vi "TestCloneAPI.vi"() -> ()   [LabVIEW 2014, in "FgenModule.lvlib"]
uses:
  FgenModule.lvlib
  TestInfo.ctl
  <userlib>/NIST/ModuleAdminLib/ModuleAdmin/ModuleAdmin.lvclass
  PublicAPI/Arguments/Broadcasts/clDidInit.ctl
  <userlib>/NIST/ModuleAdminLib/ModuleAdmin/ModuleAdmin.lvclass/ModuleAdmin.ctl
  PublicAPI/Arguments/Requests/clStopArgument.ctl
  <userlib>/NIST/ModuleAdminLib/ModuleAdmin/Accessors/Read CloneRegRef.vi
  <userlib>/NIST/ModuleAdminLib/CloneRegistration/CloneRegistration.lvclass
  FgenPlugins/FgenPluginBaseClass/FgenPluginsBase.lvclass
panel:
  in  "Reset":bool
  in  "Query ID":bool
  in  "btnInitialize":bool
  in  "btnConfigTrigs":bool
  in  "btnGetWfrms":bool
  out "Waveform Chart":waveform(dbl)[](graph)=[{"t0"=timestamp(0 s since 1904-01-01), "dt"=0.00020833333333333335, "Y"=[0.0, 0.06540312923014306, 0.13052619222005157, 0.19509032201612825, 0.25881904510252074, 0.32143946530316153, 0.3826834323650897, 0.44228869021900125, 0.49999999999999994, 0.5555702330196022, 0.6087614290087205, 0.6593458151000688, 0.7071067811865475, 0.7518398074789774, 0.793353340291235, 0.8314696123025452, 0.8660254037844385, 0.8968727415326883, 0.9238795325112866, 0.9469301294951056, 0.9659258262890682, 0.9807852804032303, 0.9914448613738104, 0.9978589232386034, 1.0, 0.9978589232386034, 0.9914448613738104, 0.9807852804032303, 0.9659258262890683, 0.9469301294951056, 0.9238795325112868, 0.8968727415326883, 0.8660254037844388, 0.8314696123025452, 0.7933533402912354, 0.7518398074789774, 0.7071067811865478, 0.6593458151000688, 0.6087614290087209, 0.5555702330196023, 0.5000000000000002, 0.4422886902190014, 0.38268343236509, 0.32143946530316175, 0.258819045102521, 0.19509032201612847, 0.13052619222005185, 0.06540312923014331, 2.669170223387751e-16, -0.06540312923014278, -0.13052619222005132, -0.19509032201612794, -0.2588190451025205, -0.32143946530316125, -0.38268343236508956, -0.4422886902190009, -0.4999999999999998, -0.5555702330196018, -0.6087614290087204, -0.6593458151000685, -0.7071067811865474, -0.751839807478977, -0.793353340291235, -0.8314696123025449, -0.8660254037844386, -0.896872741532688, -0.9238795325112867, -0.9469301294951055, -0.9659258262890683, -0.9807852804032303, -0.9914448613738105, -0.9978589232386034, -1.0, -0.9978589232386034, -0.9914448613738105, -0.9807852804032303, -0.9659258262890684, -0.9469301294951056, -0.923879532511287, -0.8968727415326883, -0.8660254037844389, -0.8314696123025452, -0.7933533402912355, -0.7518398074789775, -0.7071067811865479, -0.6593458151000691, -0.6087614290087211, -0.5555702330196025, -0.5000000000000004, -0.44228869021900163, -0.3826834323650902, -0.321439465303162, -0.25881904510252124, -0.19509032201612872, -0.13052619222005207, -0.06540312923014356]}, {"t0"=timestamp(0 s since 1904-01-01), "dt"=0.00020833333333333335, "Y"=[-0.8660254037844387, -0.8968727415326884, -0.9238795325112867, -0.9469301294951057, -0.9659258262890682, -0.9807852804032304, -0.9914448613738103, -0.9978589232386035, -0.9999999999999999, -0.9978589232386035, -0.9914448613738103, -0.9807852804032304, -0.9659258262890681, -0.9469301294951056, -0.9238795325112865, -0.8968727415326883, -0.8660254037844384, -0.8314696123025451, -0.7933533402912349, -0.7518398074789773, -0.7071067811865474, -0.6593458151000687, -0.6087614290087205, -0.5555702330196021, -0.49999999999999994, -0.44228869021900113, -0.3826834323650897, -0.3214394653031614, -0.25881904510252074, -0.1950903220161281, -0.1305261922200516, -0.06540312923014292, -4.632253781944318e-17, 0.06540312923014319, 0.13052619222005152, 0.19509032201612836, 0.25881904510252063, 0.32143946530316164, 0.3826834323650896, 0.4422886902190013, 0.49999999999999983, 0.5555702330196022, 0.6087614290087204, 0.6593458151000688, 0.7071067811865474, 0.7518398074789774, 0.7933533402912349, 0.8314696123025452, 0.8660254037844384, 0.8968727415326883, 0.9238795325112865, 0.9469301294951056, 0.9659258262890681, 0.9807852804032303, 0.9914448613738103, 0.9978589232386034, 0.9999999999999999, 0.9978589232386034, 0.9914448613738103, 0.9807852804032303, 0.9659258262890682, 0.9469301294951056, 0.9238795325112867, 0.8968727415326883, 0.8660254037844387, 0.8314696123025452, 0.7933533402912353, 0.7518398074789774, 0.7071067811865477, 0.6593458151000688, 0.6087614290087209, 0.5555702330196022, 0.5000000000000002, 0.44228869021900125, 0.38268343236509, 0.3214394653031616, 0.258819045102521, 0.1950903220161283, 0.13052619222005188, 0.06540312923014313, 3.0540619946201053e-16, -0.06540312923014296, -0.13052619222005127, -0.19509032201612814, -0.2588190451025204, -0.3214394653031614, -0.3826834323650894, -0.4422886902190011, -0.4999999999999996, -0.555570233019602, -0.6087614290087202, -0.6593458151000686, -0.7071067811865471, -0.7518398074789772, -0.7933533402912348, -0.831469612302545]}, {"t0"=timestamp(0 s since 1904-01-01), "dt"=0.00020833333333333335, "Y"=[0.8660254037844387, 0.8314696123025455, 0.7933533402912353, 0.7518398074789776, 0.7071067811865477, 0.6593458151000691, 0.6087614290087209, 0.5555702330196024, 0.5000000000000002, 0.44228869021900147, 0.38268343236509, 0.3214394653031618, 0.258819045102521, 0.19509032201612853, 0.13052619222005188, 0.06540312923014334, 3.11409968992149e-16, -0.06540312923014278, -0.13052619222005127, -0.19509032201612797, -0.2588190451025204, -0.32143946530316125, -0.3826834323650894, -0.44228869021900097, -0.4999999999999996, -0.555570233019602, -0.6087614290087202, -0.6593458151000686, -0.7071067811865471, -0.7518398074789772, -0.7933533402912348, -0.831469612302545, -0.8660254037844384, -0.8968727415326881, -0.9238795325112865, -0.9469301294951056, -0.9659258262890681, -0.9807852804032304, -0.9914448613738103, -0.9978589232386035, -0.9999999999999999, -0.9978589232386035, -0.9914448613738104, -0.9807852804032304, -0.9659258262890683, -0.9469301294951057, -0.9238795325112868, -0.8968727415326884, -0.8660254037844388, -0.8314696123025453, -0.7933533402912354, -0.7518398074789776, -0.7071067811865478, -0.6593458151000692, -0.608761429008721, -0.5555702330196026, -0.5000000000000004, -0.44228869021900175, -0.3826834323650903, -0.3214394653031621, -0.2588190451025213, -0.1950903220161288, -0.13052619222005216, -0.06540312923014363, -5.937497672345304e-16, 0.06540312923014249, 0.130526192220051, 0.1950903220161277, 0.25881904510252013, 0.32143946530316103, 0.3826834323650891, 0.44228869021900075, 0.49999999999999933, 0.5555702330196017, 0.60876142900872, 0.6593458151000684, 0.7071067811865469, 0.7518398074789769, 0.7933533402912346, 0.8314696123025448, 0.8660254037844382, 0.8968727415326879, 0.9238795325112863, 0.9469301294951054, 0.9659258262890679, 0.9807852804032302, 0.99144486137381, 0.9978589232386034, 0.9999999999999998, 0.9978589232386035, 0.9914448613738103, 0.9807852804032305, 0.9659258262890683, 0.9469301294951058, 0.9238795325112868, 0.8968727415326886]}]
  in  "btnConfigFunc":bool
  in  "btnPref":bool
  in  "btnAbortGen":bool
  in  "btnInitiateGen":bool
  in  "Show Panel":bool=TRUE
  in  "Plugin Type":u16(ring) items=["DaqMx_Single", "Single_AM", "Base Plugin", "Agilent IVI FGen", "IVI Dual FGens", "IVI FGen", "Pxi6733_AM", "Pxi6733_Sine", "Pxi6733 Sine Standalone", "PMU Cal", "Test"]
  in  "btnLoadPlugin":bool
  out "Path":path
  in  "btnRequestINIPath":bool
  in  "btnRemove":bool
  out "Status Log":string
  out "Active Modules (Array)":string[](array[string])
  in  "btnAdd":bool
  in  "btnStop":bool
  in  "Select Module":i32(ring)=-1 caption="Select Module to send Request" items=["All"=-1, "4140002"=4140002]
  # "Hidden"
  # "Visible"
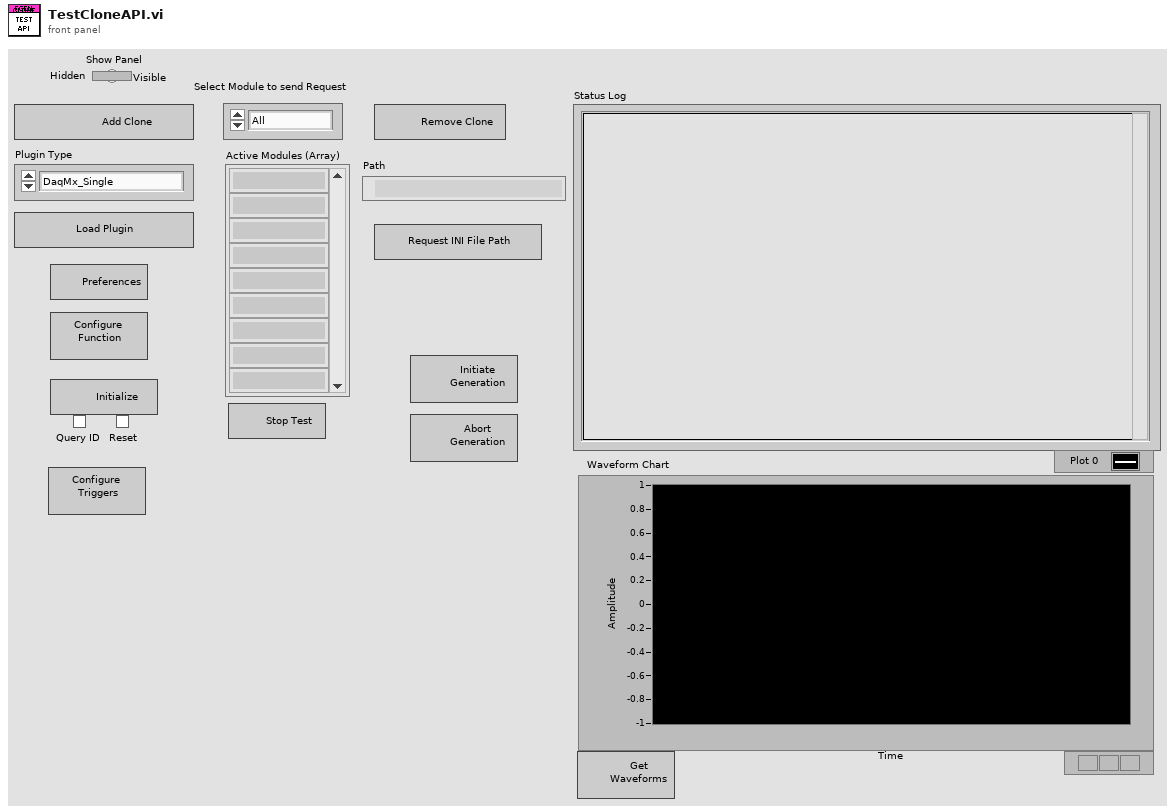
[diagram p1: front panel]
types:
  T1 = typedef "FgenModule.lvlib/TestInfo.ctl" = cluster{"PluginIniFilePaths":path[]}
  T2 = typedef "FgenModule.lvlib/clBroadcastEvents.ctl" = cluster{"DidInit":refnum<user-event>, "StatusUpdate":refnum<user-event>, "ErrorReport":refnum<user-event>, "DidStop":refnum<user-event>, "PathToINI":refnum<user-event>, "Channels":refnum<user-event>, "Function":refnum<user-event>, "Waveforms":refnum<user-event>, "Triggers":refnum<user-event>}
  T3 = typedef "FgenModule.lvlib/clDidInit.ctl" = cluster{"Init?":bool, "ModuleAdmin":refnum<class "ModuleAdmin.lvclass">}
  T4 = typedef "FgenModule.lvlib/clStopArgument.ctl" = cluster{"Exit via Stop Module Req?":bool, "Wait for Module to stop?":bool, "ModuleAdmin":refnum<class "ModuleAdmin.lvclass">}
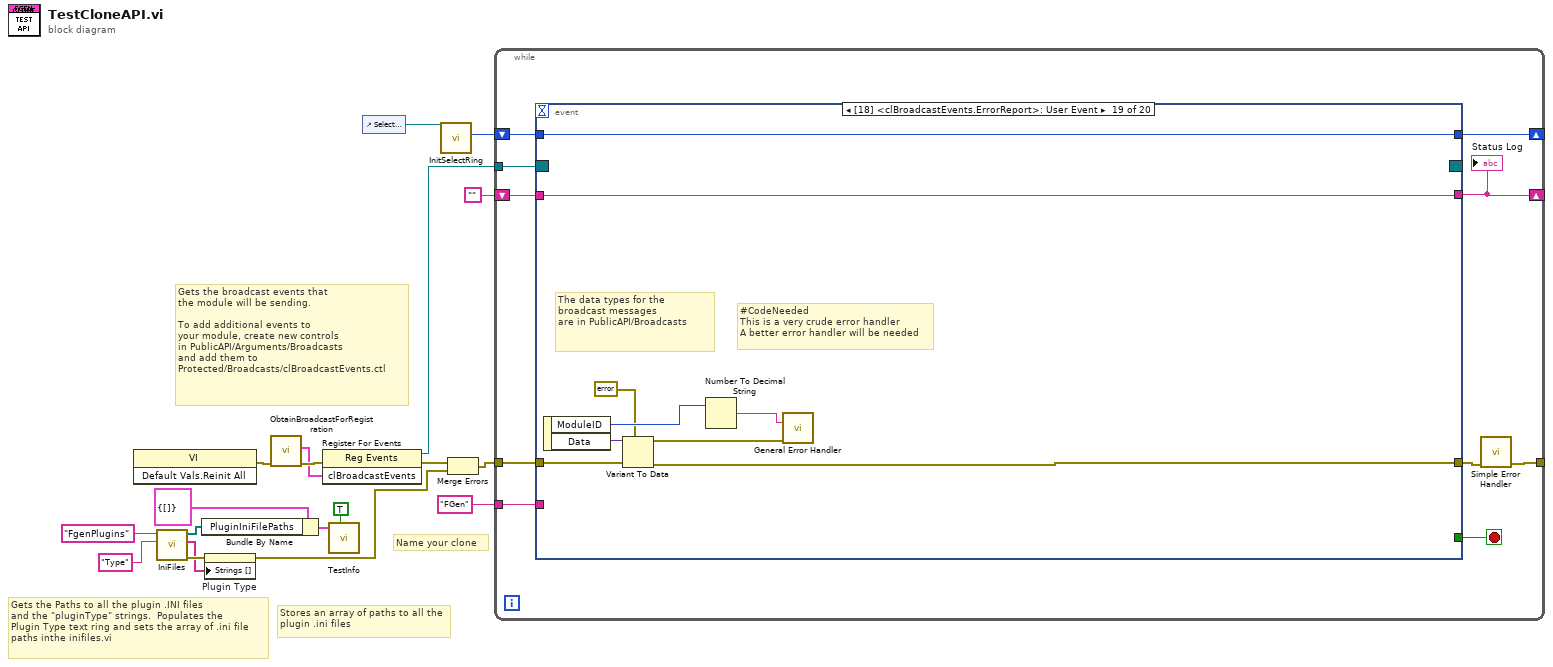
[diagram p0: block diagram]
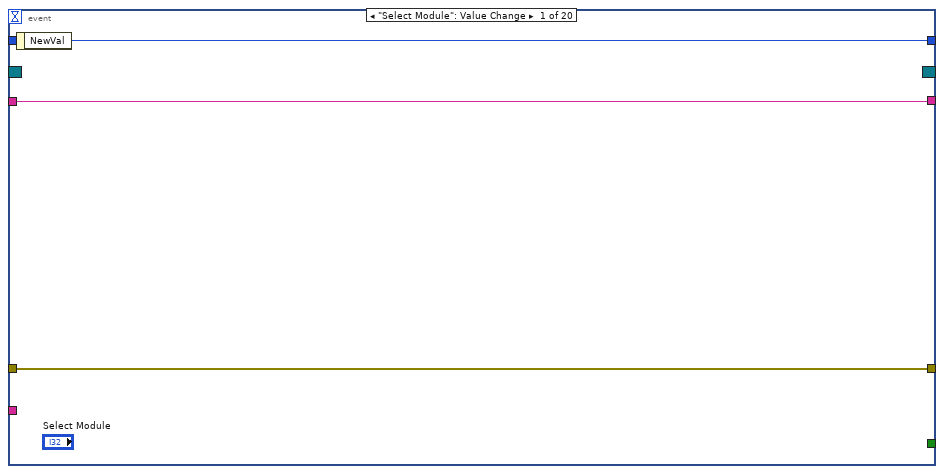
[diagram p2: hidden frame]
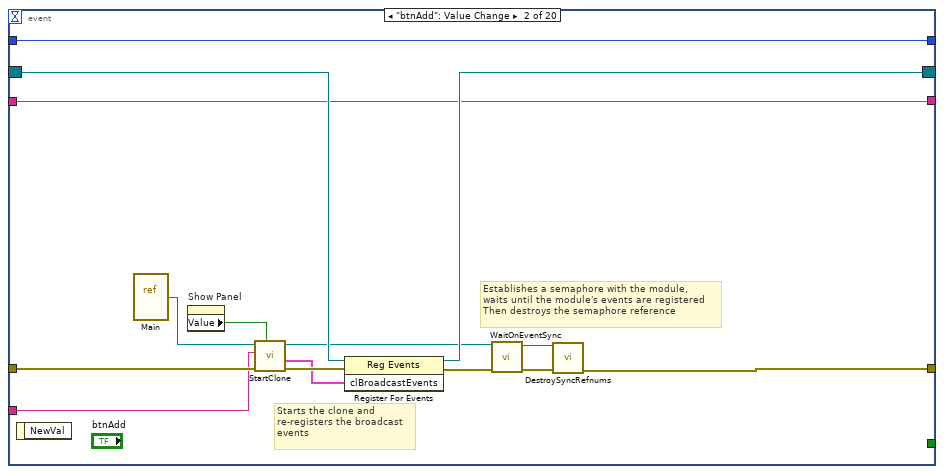
[diagram p3: hidden frame]
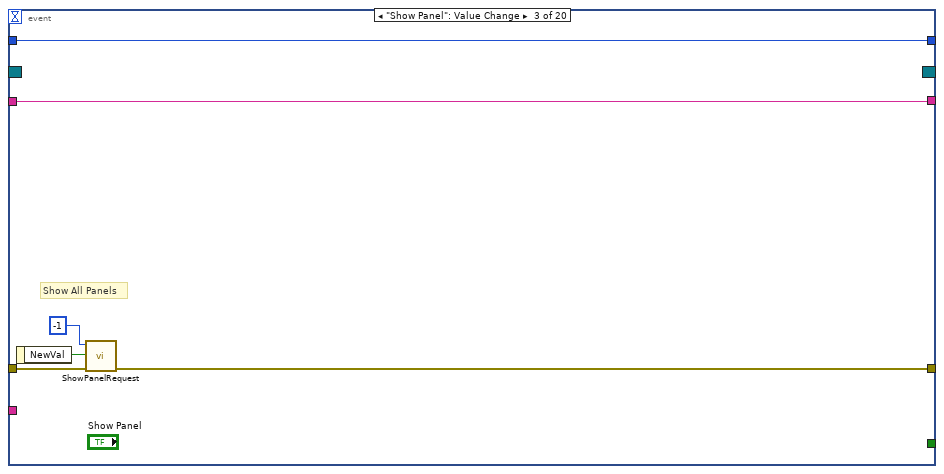
[diagram p4: hidden frame]
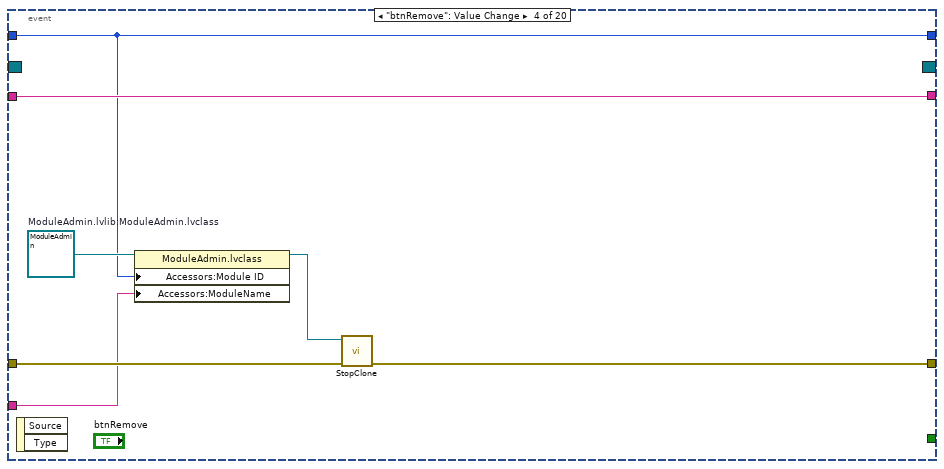
[diagram p5: hidden frame]
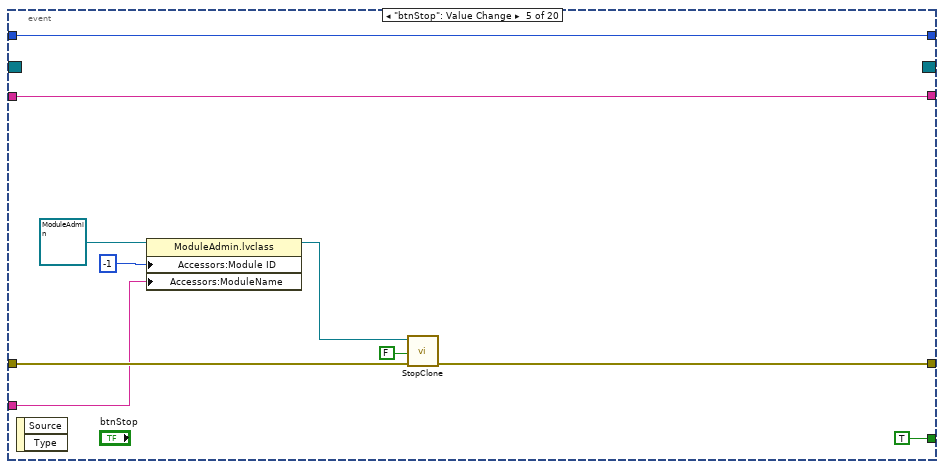
[diagram p6: hidden frame]
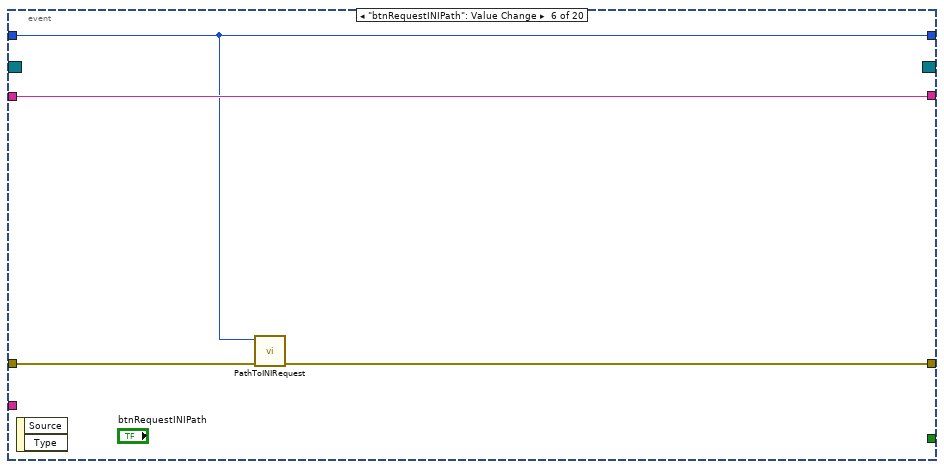
[diagram p7: hidden frame]
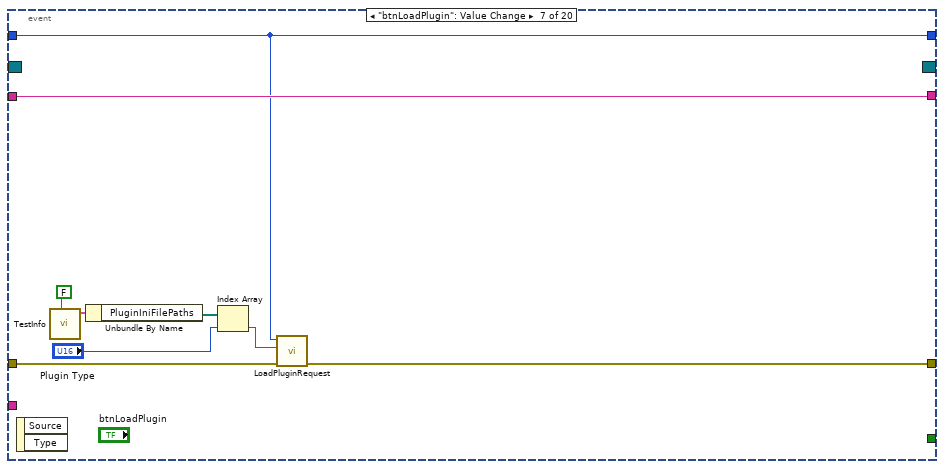
[diagram p8: hidden frame]
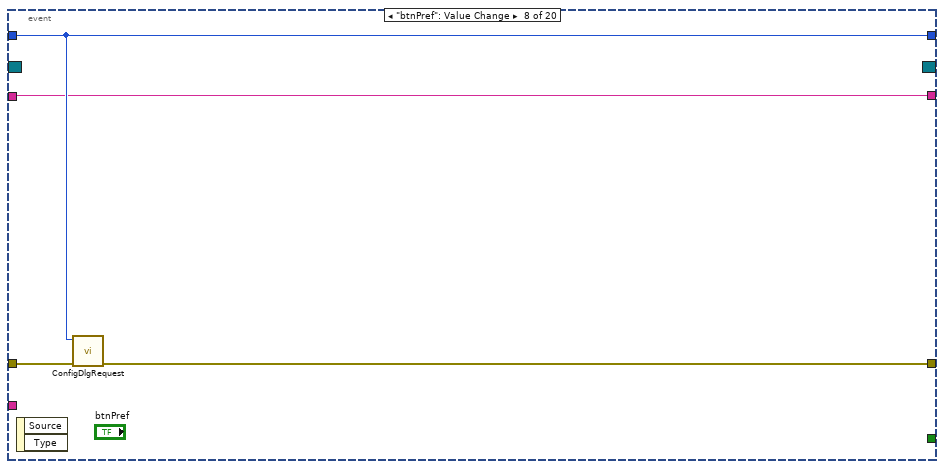
[diagram p9: hidden frame]
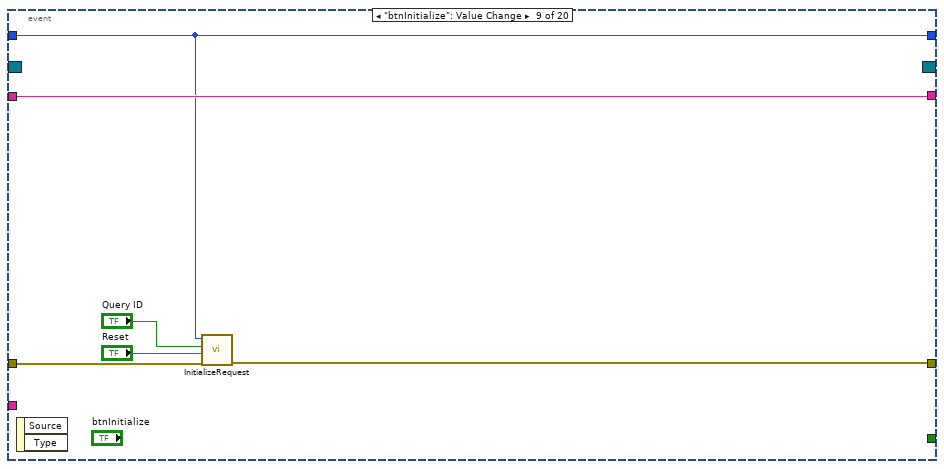
[diagram p10: hidden frame]
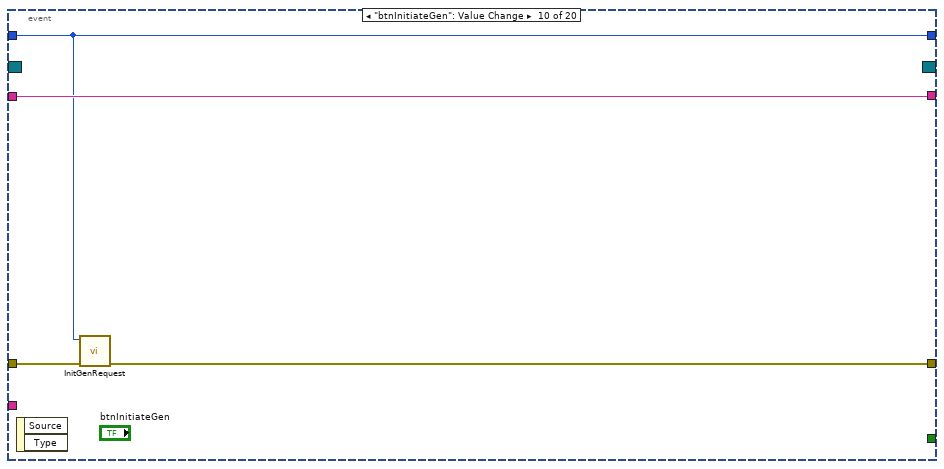
[diagram p11: hidden frame]
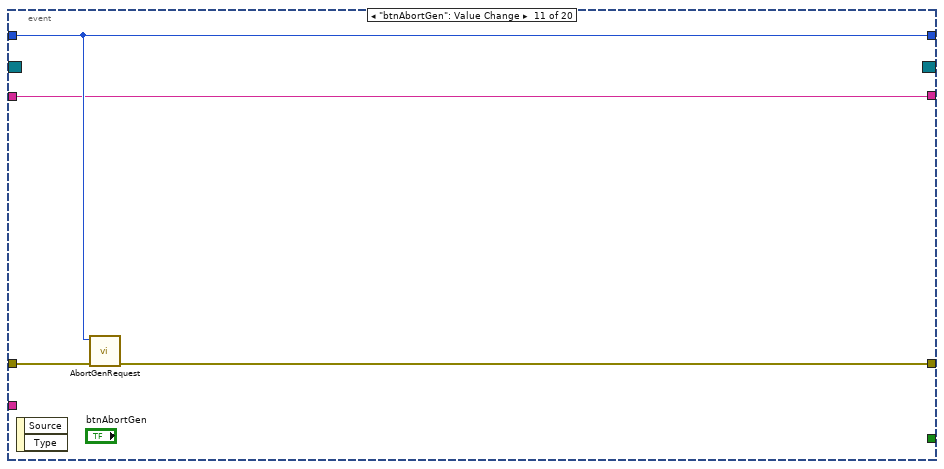
[diagram p12: hidden frame]
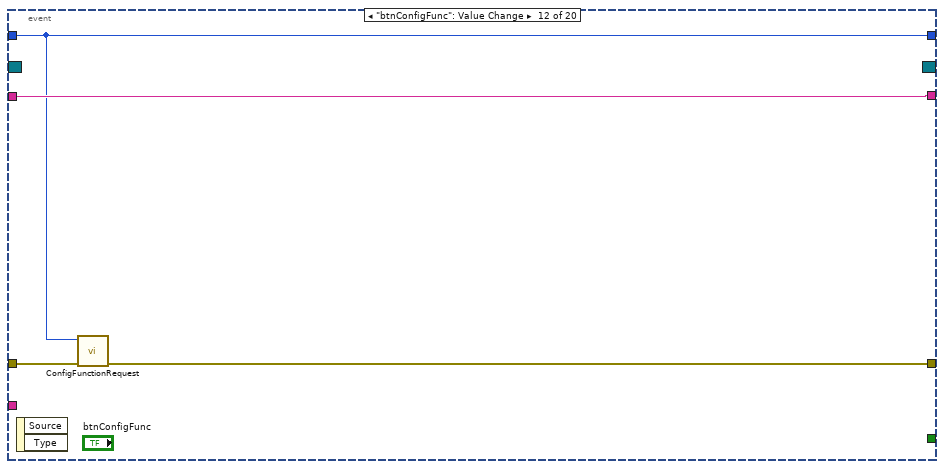
[diagram p13: hidden frame]
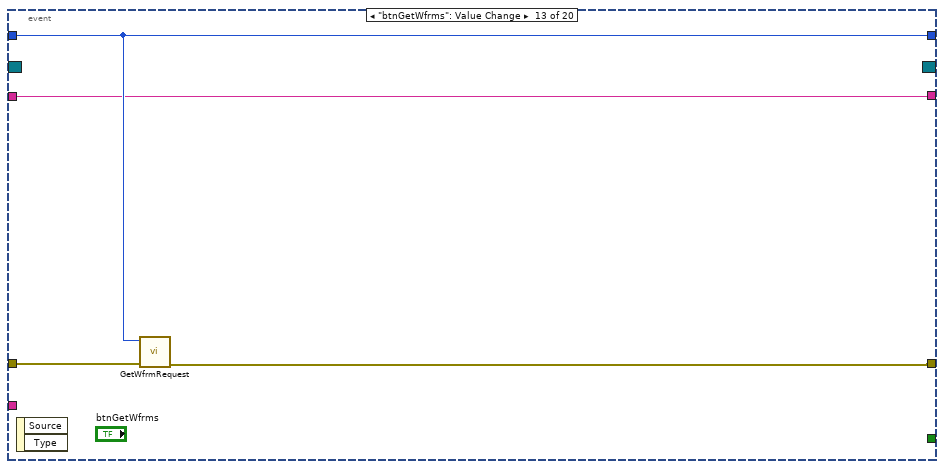
[diagram p14: hidden frame]
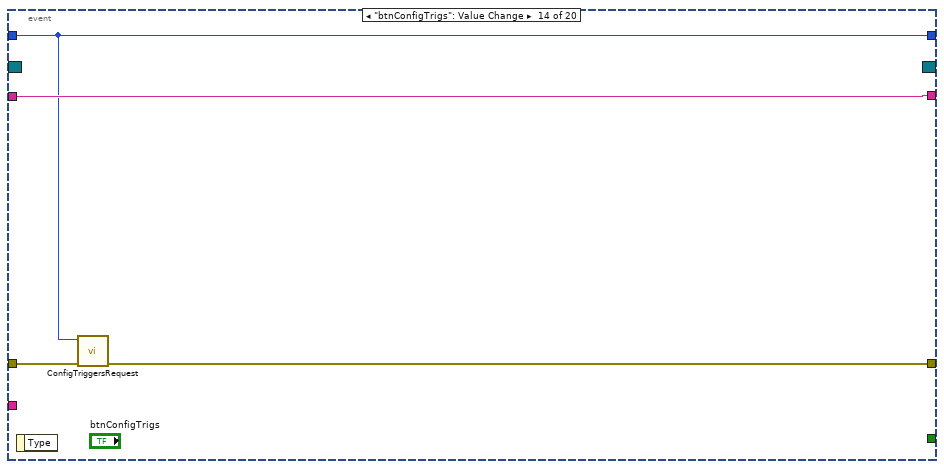
[diagram p15: hidden frame]
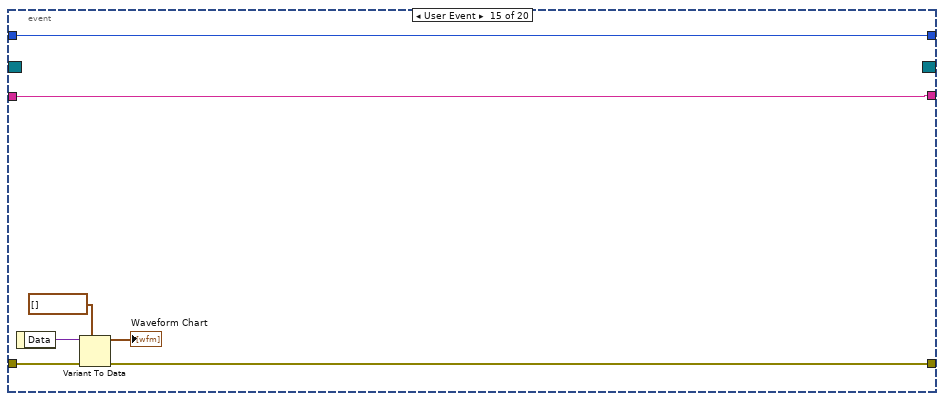
[diagram p16: hidden frame]
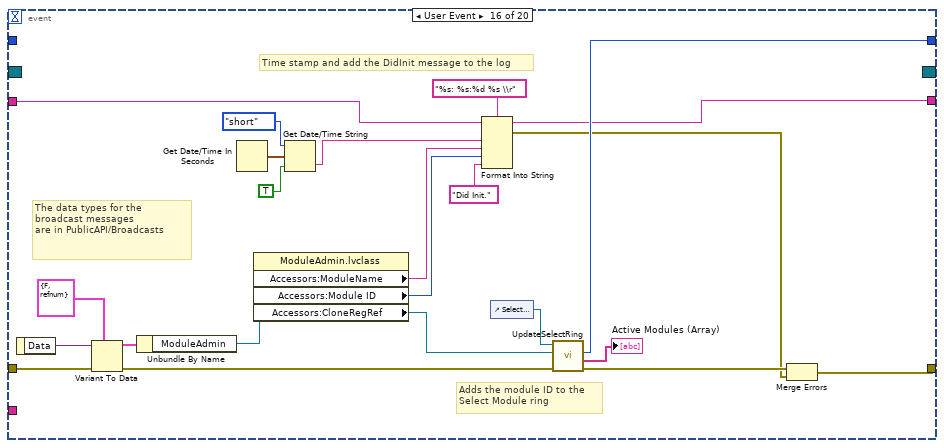
[diagram p17: hidden frame]
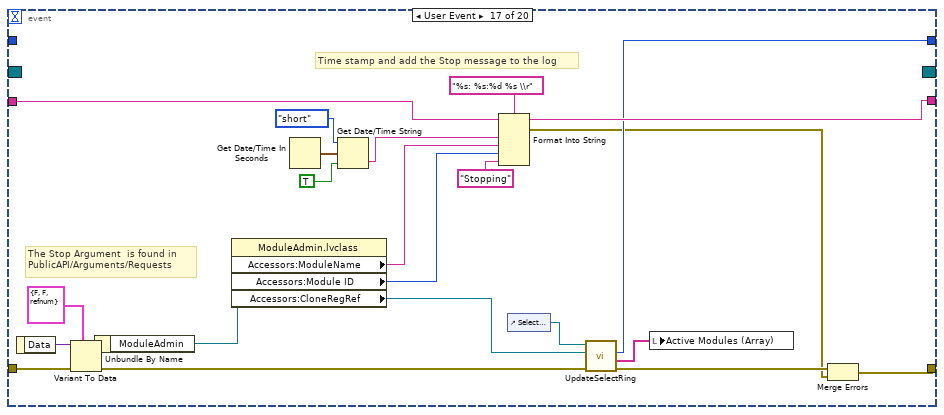
[diagram p18: hidden frame]
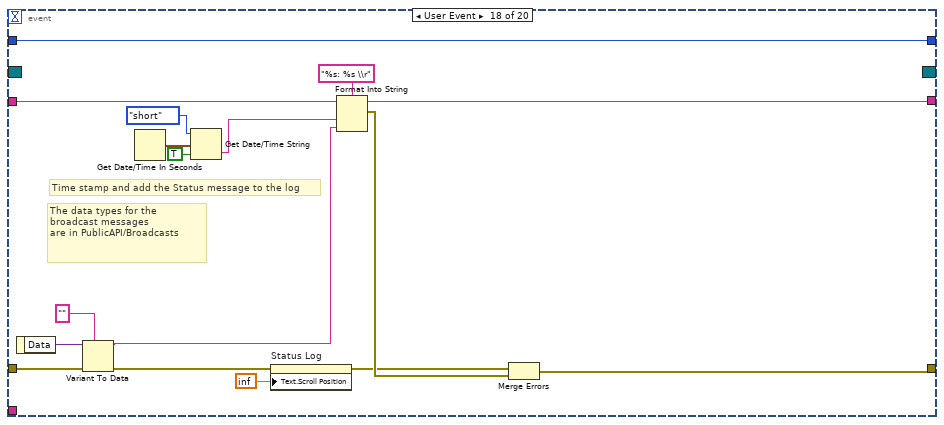
[diagram p19: hidden frame]
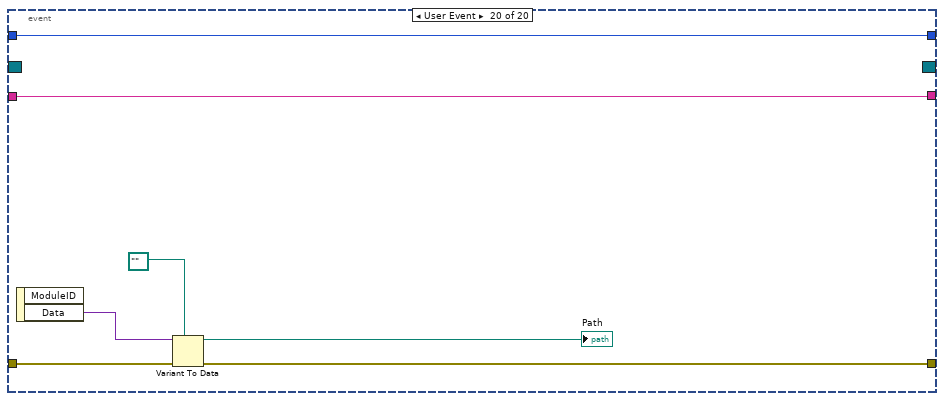
[diagram p20: hidden frame]
diagram:
  # "Stores an array of paths to all the plugin .ini files"
  # "Gets the Paths to all the plugin .INI files\nand the \"pluginType\" strings.  Populates the \nPlugin Type text ring and sets the array of .ini file\npaths inthe inifiles.vi"
  # "Name your clone"
  # "Gets the broadcast events that\nthe module will be sending.\n\nTo add additional events to\nyour module, create new controls\nin PublicAPI/Arguments/Broadcasts\nand add them to\nProtected/Broadcasts/clBroadcastEvents.ctl"
  n1 = invoke class="VI" method="Default Vals.Reinit All"() -> (error out=w17:errorcluster)  [unwired: 3 in, 2 out]
  n2 = call "IniFiles.vi"("iniKey"="Type", "name or relative path"="FgenPlugins") -> ("error out"=w10:errorcluster, "Types"=w9:string[], "IniFilePaths"=w8:path[])  [unwired: 7 in]
  n3 = Bundle By Name(cluster=T1 {"PluginIniFilePaths"=[]} ("TestInfo"), "PluginIniFilePaths"=w8) -> (w7:T1)
  n4 = property on="Plugin Type" class="Ring (strict)"(error in=w10, "Strings []"=w9) -> (error out=w4:errorcluster)  [unwired: 1 in, 1 out]
  n5 = call "ObtainBroadcastForRegistration.vi"("error in (no error)"=w17) -> ("error out"=w16:errorcluster, "clBroadcastEvents"=w15:T2)  [unwired: 9 in]
  n6 = register-events(error in=w16, w15) -> (reference out=w13:refnum<event-registration>, error out=w14:errorcluster)  [unwired: 1 in]
  n7 = call "TestInfo.vi"("Set (f)"=TRUE, "TestInfo 2"=w7) -> ()  [unwired: 9 in, 1 out]
  n8 = control-ref of="Select Module"() -> (w19:refnum<vi>)
  n9 = call "InitSelectRing.vi"("Ring Refnum"=w19) -> ("Module Ring Value"=w18:i32)  [unwired: 9 in, 1 out]
  n10 = Merge Errors(w14, w4) -> (w5:errorcluster)
  n11 = while {
    shift-right: [w28] -> _
    shift-left: w18 -> [w29]
    tunnel: w5 -> [w26]
    tunnel: w13 -> [w23]
    tunnel: [w24] -> _
    shift-right: [w22] -> _
    shift-left: "" -> [w21]
    tunnel: "FGen" ("ModuleName") -> [w20]
    stop <- w27 stop-if-true
    n12 = event shown="[18] <clBroadcastEvents.ErrorReport>: User Event" {
      selector: w23 -> [_ w39 _ _ _ _ _ _ _ _ _ _ _ _ _ _ _ _ _ _]
      dyn-events: [_ w38 _ _ _ _ _ _ _ _ _ _ _ _ _ _ _ _ _ _] -> _
      timeout: _ -> [_ _ _ _ _ _ _ _ _ _ _ _ _ _ _ _ _ _ _ _]
      tunnel: w29 -> [_ w47 w49 w56 w70 w73 w76 w86 w89 w95 w100 w103 w108 w111 w114 _ _ w183 w187 w198]
      tunnel: [w32 w47 w49 w56 w70 w73 w76 w86 w89 w95 w100 w103 w108 w111 w114 w138 w153 w183 w187 w198] -> w28
      tunnel: [_ _ _ _ TRUE _ _ _ _ _ _ _ _ _ _ _ _ _ _ _] -> w27
      tunnel: w26 -> [w30 w46 w52 w59 w68 w72 w82 w87 w92 w97 w101 w104 w109 w113 w119 w143 w162 w180 w191 w194]
      tunnel: [w30 w40 w50 w58 w66 w71 w75 w84 w88 w94 w98 w102 w106 w110 w116 w127 w150 w175 w190 w193] -> w25
      tunnel: [w31 w36 w48 w60 w65 w74 w83 w85 w93 w96 w99 w105 w107 w112 w115 w131 w159 w177 w186 w199] -> w22
      tunnel: w21 -> [w31 w36 w48 w60 w65 w74 w83 w85 w93 w96 w99 w105 w107 w112 w115 w130 w160 w182 w186 w199]
      tunnel: w20 -> [_ w35 _ w55 w62 _ _ _ _ _ _ _ _ _ _ _ _ _ _ _]
      event "Select Module": Value Change {
        n13 = event-data() -> ("NewVal"=w32:i32)  [unwired: 1 in]
      }
      event "btnAdd": Value Change {
        # "Establishes a semaphore with the module,\nwaits until the module's events are registered\nThen destroys the semaphore reference"
        # "Starts the clone and\nre-registers the broadcast \nevents"
        n14 = event-data() -> ()  [unwired: 1 in, 1 out]
        n15 = vi-ref "Main.vi"() -> (w37:refnum<vi>)
        n16 = property on="Show Panel" class="Bool (strict)"() -> ("Value"=w33:bool)  [unwired: 2 in, 2 out]
        n17 = call "StartClone.vi"("ShowPanel? (f)"=w33, "error in (no error)"=w46, "ModuleName"=w35, "VI Refnum"=w37) -> ("error out"=w45:errorcluster, "clBroadcastEvents"=w41:T2, "ModuleAdmin"=w34:refnum<class "ModuleAdmin.lvclass">)  [unwired: 5 in]
        n18 = register-events(reference=w39, error in=w45, w41) -> (reference out=w38:refnum<event-registration>, error out=w44:errorcluster)
        n19 = call <userlib>:"WaitOnEventSync.vi"("error in (no error)"=w44, "ModuleAdmin"=w34) -> ("error out"=w43:errorcluster, "ModuleAdmin"=w42:refnum<class "ModuleAdmin.lvclass">)  [unwired: 8 in]
        n20 = call <userlib>:"DestroySyncRefnums.vi"("error in (no error)"=w43, "ModuleAdmin"=w42) -> ("error out"=w40:errorcluster)  [unwired: 9 in]
      }
      event "Show Panel": Value Change {
        # "Show All Panels"
        n21 = event-data() -> ("NewVal"=w53:bool)  [unwired: 1 in]
        n22 = call "ShowPanelRequest.vi"("error in (no error)"=w52, "ShowPanel?"=w53, "ModuleID"=-1) -> ("error out"=w50:errorcluster)  [unwired: 8 in]
      }
      event "btnRemove": Value Change {
        w57 = refnum<class "ModuleAdmin.lvclass"> refnum  # ModuleAdmin.lvlib:ModuleAdmin.lvclass
        n23 = event-data() -> ()  [unwired: 1 in, 2 out]
        n24 = property class="ModuleAdmin.lvclass"(reference=w57, "Accessors:Module ID"=w56, "Accessors:ModuleName"=w55) -> (reference out=w54:refnum<class "ModuleAdmin.lvclass">)  [unwired: 1 in, 1 out]
        n25 = call "StopClone.vi"("error in (no error)"=w59, "ModuleAdmin"=w54) -> ("error out"=w58:errorcluster)  [unwired: 9 in]
      }
      event "btnStop": Value Change {
        n26 = event-data() -> ()  [unwired: 1 in, 2 out]
        n27 = property class="ModuleAdmin.lvclass"(reference=refnum<class "ModuleAdmin.lvclass"> refnum ("ModuleAdmin.lvlib:ModuleAdmin.lvclass"), "Accessors:Module ID"=-1 ("Module ID"), "Accessors:ModuleName"=w62) -> (reference out=w61:refnum<class "ModuleAdmin.lvclass">)  [unwired: 1 in, 1 out]
        n28 = call "StopClone.vi"("error in (no error)"=w68, "Wait for Module to stop?"=FALSE, "ModuleAdmin"=w61) -> ("error out"=w66:errorcluster)  [unwired: 8 in]
      }
      event "btnRequestINIPath": Value Change {
        n29 = event-data() -> ()  [unwired: 1 in, 2 out]
        n30 = call "PathToINIRequest.vi"("error in (no error)"=w72, "ModuleID"=w73) -> ("error out"=w71:errorcluster)  [unwired: 9 in]
      }
      event "btnLoadPlugin": Value Change {
        n31 = event-data() -> ()  [unwired: 1 in, 2 out]
        n32 = call "TestInfo.vi"("Set (f)"=FALSE) -> ("TestInfo"=w80:T1)  [unwired: 10 in]
        n33 = Unbundle By Name(w80) -> ("PluginIniFilePaths"=w79:path[])
        n34 = Index Array(array=w79, index="Plugin Type") -> (element=w77:path)
        n35 = call "LoadPluginRequest.vi"("error in (no error)"=w82, "PathToPluginINI"=w77, "ModuleID"=w76) -> ("error out"=w75:errorcluster)  [unwired: 8 in]
      }
      event "btnPref": Value Change {
        n36 = event-data() -> ()  [unwired: 1 in, 2 out]
        n37 = call "ConfigDlgRequest.vi"("error in (no error)"=w87, "ModuleID"=w86) -> ("error out"=w84:errorcluster)  [unwired: 9 in]
      }
      event "btnInitialize": Value Change {
        n38 = event-data() -> ()  [unwired: 1 in, 2 out]
        n39 = call "InitializeRequest.vi"("error in (no error)"=w92, "Reset"="Reset", "IDQuery"="Query ID", "ModuleID"=w89) -> ("error out"=w88:errorcluster)  [unwired: 7 in]
      }
      event "btnInitiateGen": Value Change {
        n40 = event-data() -> ()  [unwired: 1 in, 2 out]
        n41 = call "InitGenRequest.vi"("error in (no error)"=w97, "ModuleID"=w95) -> ("error out"=w94:errorcluster)  [unwired: 9 in]
      }
      event "btnAbortGen": Value Change {
        n42 = event-data() -> ()  [unwired: 1 in, 2 out]
        n43 = call "AbortGenRequest.vi"("error in (no error)"=w101, "ModuleID"=w100) -> ("error out"=w98:errorcluster)  [unwired: 9 in]
      }
      event "btnConfigFunc": Value Change {
        n44 = event-data() -> ()  [unwired: 1 in, 2 out]
        n45 = call "ConfigFunctionRequest.vi"("error in (no error)"=w104, "ModuleID"=w103) -> ("error out"=w102:errorcluster)  [unwired: 9 in]
      }
      event "btnGetWfrms": Value Change {
        n46 = event-data() -> ()  [unwired: 1 in, 2 out]
        n47 = call "GetWfrmRequest.vi"("error in (no error)"=w109, "ModuleID"=w108) -> ("error out"=w106:errorcluster)  [unwired: 9 in]
      }
      event "btnConfigTrigs": Value Change {
        n48 = event-data() -> ()  [unwired: 1 in, 1 out]
        n49 = call "ConfigTriggersRequest.vi"("error in (no error)"=w113, "ModuleID"=w111) -> ("error out"=w110:errorcluster)  [unwired: 9 in]
      }
      event User Event {
        n50 = event-data() -> ("Data"=w120:variant)  [unwired: 1 in]
        n51 = Variant To Data(error in=w119, type=waveform(dbl)[] [] ("Waveforms"), Variant=w120) -> (data=→"Waveform Chart":waveform(dbl)[], error out=w116:errorcluster)
      }
      event User Event {
        # "Adds the module ID to the \nSelect Module ring"
        # "Time stamp and add the DidInit message to the log"
        # "The data types for the broadcast messages\nare in PublicAPI/Broadcasts"
        n52 = event-data() -> ("Data"=w142:variant)  [unwired: 1 in]
        n53 = Variant To Data(error in=w143, type=T3 {"Init?"=FALSE, "ModuleAdmin"=refnum} ("clDidInit"), Variant=w142) -> (data=w135:T3, error out=w140:errorcluster)
        n54 = Unbundle By Name(w135) -> ("ModuleAdmin"=w125:refnum<class "ModuleAdmin.lvclass">)
        n55 = Get Date/Time In Seconds() -> (seconds since 1Jan1904=w133:timestamp)
        n56 = property class="ModuleAdmin.lvclass"(reference=w125) -> ("Accessors:ModuleName"=w123:string, "Accessors:Module ID"=w122:i32, "Accessors:CloneRegRef"=w121:refnum<data-value>)  [unwired: 1 in, 2 out]
        n57 = Get Date/Time String(date format (0)=enum16{"short", "long", "abbreviated"}."short", seconds (now)=w133, want seconds? (F)=TRUE) -> (time string=w136:string)  [unwired: 1 out]
        n58 = Format Into String(format string="%s: %s:%d %s \\r", initial string=w130, w136, w123, w122, "Did Init.") -> (resulting string=w131:string, error out=w128:errorcluster)  [unwired: 1 in]
        n59 = control-ref of="Select Module"() -> (w139:refnum<vi>)
        n60 = call "UpdateSelectRing.vi"("error in (no error)"=w140, "CloneRegRef"=w121, "Ring Refnum"=w139) -> ("error out"=w129:errorcluster, "ActiveModules"=→"Active Modules (Array)":string[], "Module Ring Value"=w138:i32)  [unwired: 6 in]
        n61 = Merge Errors(w129, w128) -> (w127:errorcluster)
      }
      event User Event {
        # "Time stamp and add the Stop message to the log"
        # "The Stop Argument  is found in\nPublicAPI/Arguments/Requests"
        n62 = event-data() -> ("Data"=w161:variant)  [unwired: 1 in]
        n63 = Variant To Data(error in=w162, type=T4 {"Exit via Stop Module Req?"=FALSE, "Wait for Module to stop?"=FALSE, "ModuleAdmin"=refnum} ("Stop Argument"), Variant=w161) -> (data=w157:T4, error out=w156:errorcluster)
        n64 = Unbundle By Name(w157) -> ("ModuleAdmin"=w148:refnum<class "ModuleAdmin.lvclass">)
        n65 = property class="ModuleAdmin.lvclass"(reference=w148) -> ("Accessors:ModuleName"=w146:string, "Accessors:Module ID"=w145:i32, "Accessors:CloneRegRef"=w144:refnum<data-value>)  [unwired: 1 in, 2 out]
        n66 = Get Date/Time In Seconds() -> (seconds since 1Jan1904=w164:timestamp)
        n67 = Get Date/Time String(date format (0)=enum16{"short", "long", "abbreviated"}."short", seconds (now)=w164, want seconds? (F)=TRUE) -> (time string=w166:string)  [unwired: 1 out]
        n68 = Format Into String(format string="%s: %s:%d %s \\r", initial string=w160, w166, w146, w145, "Stopping") -> (resulting string=w159:string, error out=w151:errorcluster)  [unwired: 1 in]
        n69 = control-ref of="Select Module"() -> (w155:refnum<vi>)
        n70 = call "UpdateSelectRing.vi"("error in (no error)"=w156, "CloneRegRef"=w144, "Ring Refnum"=w155) -> ("error out"=w152:errorcluster, "ActiveModules"=w154:string[], "Module Ring Value"=w153:i32)  [unwired: 6 in]
        n71 = local write "Active Modules (Array)"(w154) -> ()
        n72 = Merge Errors(w152, w151) -> (w150:errorcluster)
      }
      event User Event {
        # "Time stamp and add the Status message to the log"
        # "The data types for the broadcast messages\nare in PublicAPI/Broadcasts"
        n73 = event-data() -> ("Data"=w179:variant)  [unwired: 1 in]
        n74 = Variant To Data(error in=w180, type="", Variant=w179) -> (data=w167:string, error out=w171:errorcluster)
        n75 = Get Date/Time In Seconds() -> (seconds since 1Jan1904=w178:timestamp)
        n76 = Get Date/Time String(date format (0)=enum16{"short", "long", "abbreviated"}."short", seconds (now)=w178, want seconds? (F)=TRUE) -> (time string=w172:string)  [unwired: 1 out]
        n77 = property on="Status Log" class="Str"(error in=w171, "Text.Scroll Position"=inf) -> (error out=w170:errorcluster)  [unwired: 1 in, 1 out]
        n78 = Format Into String(format string="%s: %s \\r", initial string=w182, w172, w167) -> (resulting string=w177:string, error out=w176:errorcluster)  [unwired: 1 in]
        n79 = Merge Errors(w170, w176) -> (w175:errorcluster)
      }
      event User Event {
        # "#CodeNeeded\nThis is a very crude error handler\nA better error handler will be needed"
        # "The data types for the broadcast messages\nare in PublicAPI/Broadcasts"
        n80 = event-data() -> ("ModuleID"=w189:i32, "Data"=w192:variant)  [unwired: 1 in]
        n81 = Variant To Data(error in=w191, type=errorcluster {"status"=FALSE, "code"=0, "source"=""} ("error constant"), Variant=w192) -> (data=w184:errorcluster, error out=w190:errorcluster)
        n82 = Number To Decimal String(number=w189) -> (decimal integer string=w188:string)  [unwired: 1 in]
        n83 = call <vilib>:"General Error Handler.vi"("[error source] (\" \")"=w188, "error in (no error)"=w184) -> ()  [unwired: 9 in, 5 out]
      }
      event User Event {
        n84 = event-data() -> ("Data"=w196:variant)  [unwired: 1 in, 1 out]
        n85 = Variant To Data(error in=w194, type=path "" ("Path"), Variant=w196) -> (data=→"Path":path, error out=w193:errorcluster)
      }
    }
    "Status Log" <- w22
    n86 = call <vilib>:"Simple Error Handler.vi"("error in (no error)"=w25) -> ("error out"=w24:errorcluster)  [unwired: 4 in, 4 out]
  }
